vi "RemoveBTDevices.vi"(8 "error in (no error)":errorcluster caption="错误输入（无错误）") -> (0 "error out":errorcluster caption="错误输出")   [LabVIEW 2013]
uses:
  GlobalValue.vi
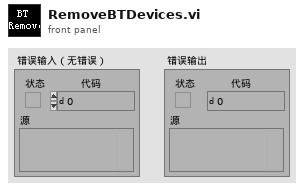
[diagram p1: front panel]
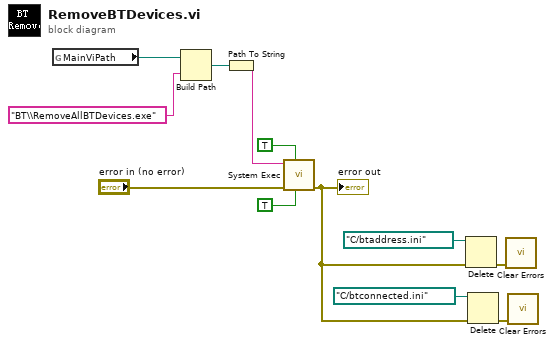
[diagram p0: block diagram]
diagram:
  n1 = global read "GlobalValue.vi" "MainViPath"() -> (w4:path)
  n2 = Build Path(base path=w4, name or relative path="BT\\RemoveAllBTDevices.exe" ("command line")) -> (appended path=w11:path)
  n3 = Path To String(path=w11) -> (string=w9:string)
  n4 = call <vilib>:"System Exec.vi"("run minimized? (F)"=TRUE, "wait until completion? (T)"=TRUE, "error in (no error)"="error in (no error)", "command line"=w9) -> ("error out"=w1:errorcluster)  [unwired: 4 in, 3 out]
  "error out" <- w1
  n5 = Delete(path (use dialog)=path "C:/btaddress.ini" ("路径（使用对话框）"), error in=w1) -> (error out=w5:errorcluster)  [unwired: 3 in, 2 out]
  n6 = Delete(path (use dialog)=path "C:/btconnected.ini" ("路径（使用对话框）"), error in=w1) -> (error out=w3:errorcluster)  [unwired: 3 in, 2 out]
  n7 = call <vilib>:"Clear Errors.vi"("error in (no error)"=w5) -> ()  [unwired: 6 in, 1 out]
  n8 = call <vilib>:"Clear Errors.vi"("error in (no error)"=w3) -> ()  [unwired: 6 in, 1 out]
